vi "Reset.vi"(8 "error in (no error)":errorcluster, 10 "Name":string, 11 "BCAdmin":refnum<class "BCAdmin.lvclass">) -> (0 "error out":errorcluster, 3 "BCAdmin 2":refnum<class "BCAdmin.lvclass">)   [LabVIEW 2017, in "BusController.lvlib" / "BCAdmin.lvclass"]
uses:
  BCAdmin.lvclass
  BCAdmin.lvclass/BCAdmin.ctl
  Accessors/Write BC ID.vi
  Accessors/Write First_.vi
  Accessors/Write Name.vi
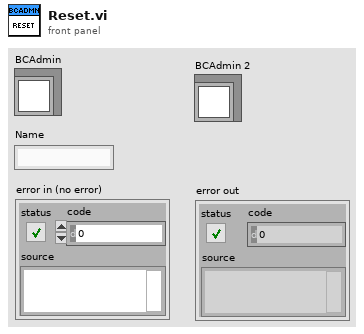
[diagram p1: front panel]
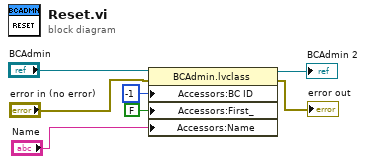
[diagram p0: block diagram]
diagram:
  n1 = property class="BCAdmin.lvclass"(reference="BCAdmin", error in="error in (no error)", "Accessors:BC ID"=-1 ("BC ID"), "Accessors:First_"=FALSE ("First_"), "Accessors:Name"="Name") -> (reference out=→"BCAdmin 2":refnum<class "BCAdmin.lvclass">, error out=→"error out":errorcluster)
